vi "FFT_impl (SubVI).vi"(11 "Array":dbl[](array[numeric])) -> (3 "FFT{x}":cdb[](array[numeric]))   [LabVIEW 2025]
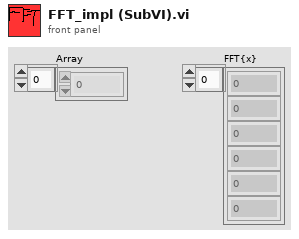
[diagram p1: front panel]
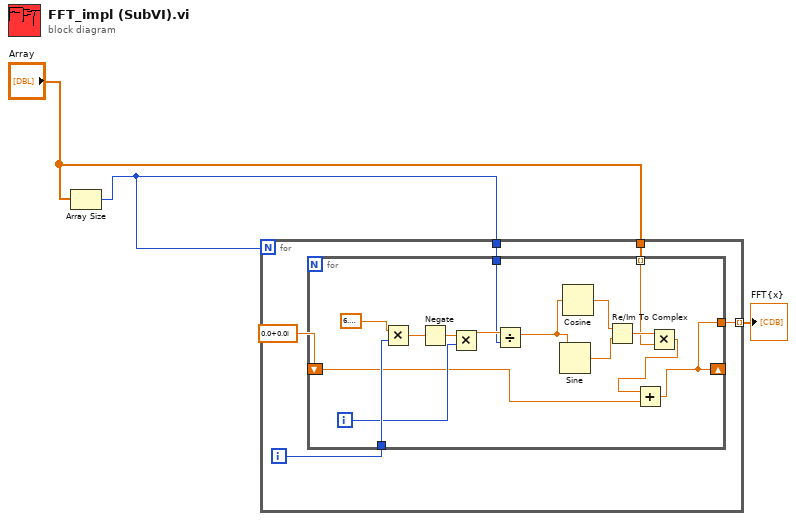
[diagram p0: block diagram]
diagram:
  n1 = Array Size(array="Array") -> (size(s)=w3:i32)
  n2 = for {
    N: w3 -> [_]
    tunnel: w3 -> [w7]
    tunnel: "Array" -> [w6]
    tunnel: [w4] -> w2 mode=indexing
    i -> [w8]
    n3 = for {
      tunnel: w8 -> [w21]
      tunnel: w7 -> [w17]
      tunnel: w6 -> [w12] mode=indexing
      shift-right: [w9] -> _
      shift-left: cdb 0.0+0.0i -> [w11]
      tunnel: [w9] -> w4
      i -> [w19]
      n4 = Multiply(x=6.283185307179586, y=w21) -> (x*y=w22:dbl)
      n5 = Negate(x=w22) -> (-x=w20:dbl)
      n6 = Multiply(x=w20, y=w19) -> (x*y=w18:dbl)
      n7 = Divide(x=w18, y=w17) -> (x/y=w16:dbl)
      n8 = Sine(x=w16) -> (sin(x)=w14:dbl)
      n9 = Cosine(x=w16) -> (cos(x)=w15:dbl)
      n10 = Re/Im To Complex(1:w14, 2:w15) -> (0:w13:cdb)
      n11 = Multiply(x=w13, y=w12) -> (x*y=w10:cdb)
      n12 = Add(x=w10, y=w11) -> (x+y=w9:cdb)
    }
  }
  "FFT{x}" <- w2
